vi "formulanode.vi"() -> ()   [LabVIEW 2025]
panel:
  out "Boolean":bool
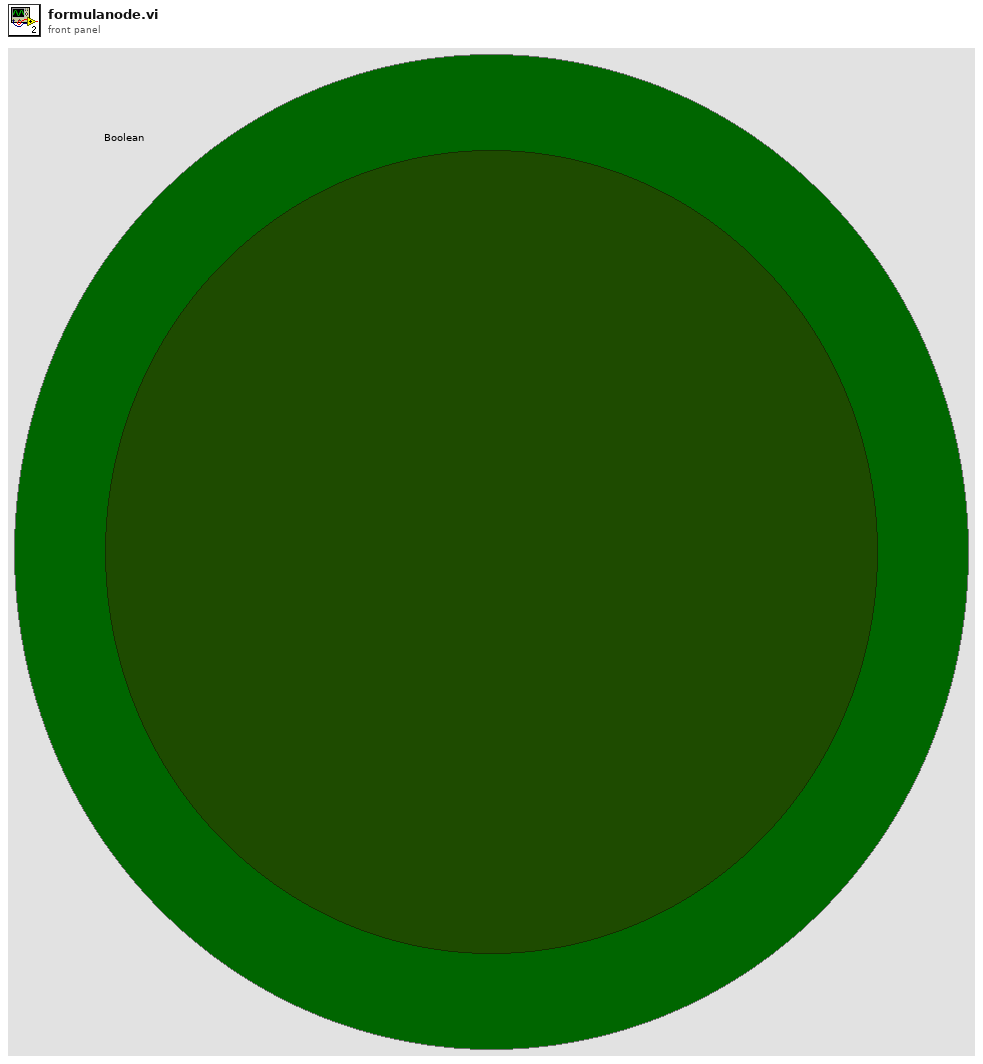
[diagram p1: front panel]
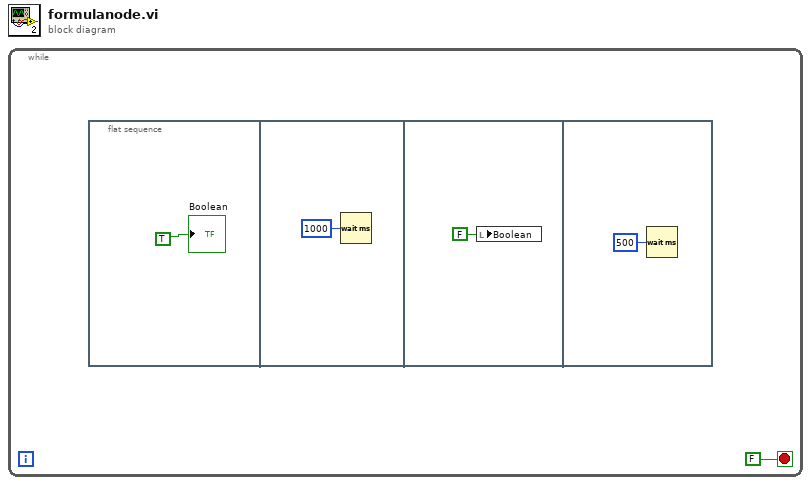
[diagram p0: block diagram]
diagram:
  n1 = while {
    stop <- FALSE stop-if-true
    n2 = flat-sequence {
      frame #0 {
        "Boolean" <- TRUE ("Boolean 2")
      }
      frame #1 {
        n3 = Wait (ms)(milliseconds to wait=u32 1000) -> ()  [unwired: 1 out]
      }
      frame #2 {
        n4 = local write "Boolean"(FALSE ("Boolean")) -> ()
      }
      frame #3 {
        n5 = Wait (ms)(milliseconds to wait=u32 500) -> ()  [unwired: 1 out]
      }
    }
  }
